vi "Database.File.Move.vi"(8 "error in (no error)":errorcluster, 10 "FileBody":T1 {"Values" format="%.3f"}) -> (0 "error out":errorcluster)   [LabVIEW 2016]
uses:
  Global/ApplicationGlobal.vi
  Logger/Logger.FileBody.ctl
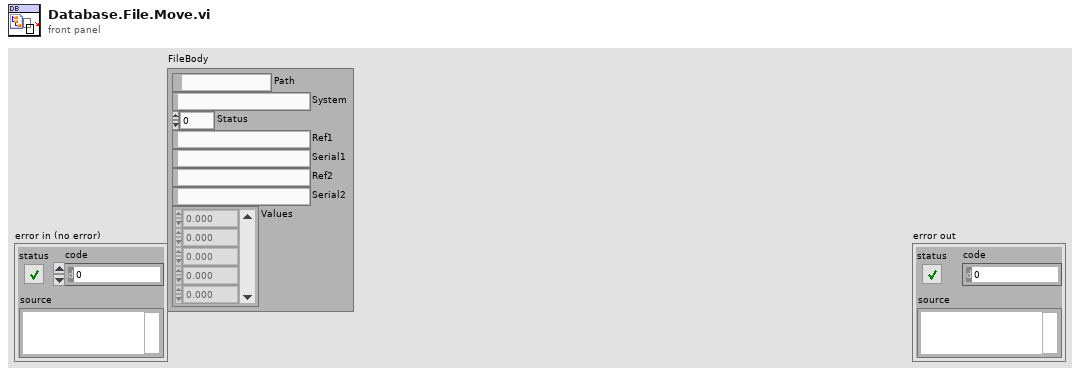
[diagram p1: front panel]
types:
  T1 = typedef "Logger.FileBody.ctl" = cluster{"Path":path, "System":string, "Status":u8, "Ref1":string, "Serial1":string, "Ref2":string, "Serial2":string, "Values":sgl[]}
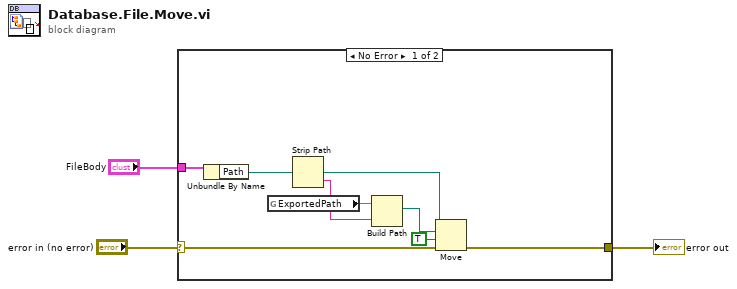
[diagram p0: block diagram]
diagram:
  n1 = case shown="No Error" "error in (no error)" {
    selector: "error in (no error)" -> [w6 w12]
    tunnel: "FileBody" -> [w11 _]
    tunnel: [w5 w12] -> w1
    frame No Error {
      n2 = Unbundle By Name(w11) -> ("Path"=w8:path)
      n3 = global read "ApplicationGlobal.vi" "ExportedPath"() -> (w10)
      n4 = Strip Path(path=w8) -> (name=w9:string)  [unwired: 1 out]
      n5 = Build Path(base path=w10, name or relative path=w9) -> (appended path=w7:path)
      n6 = Move(source path=w8, error in=w6, 9:TRUE ("overwrite (F)"), 10:w7) -> (error out=w5:errorcluster)  [unwired: 1 in, 2 out]
    }
    frame Error {
    }
  }
  "error out" <- w1
